vi "Write Value.vi"(8 "error in (no error)":errorcluster, 10 "Value":i64, 11 "int32 in":refnum<class "int64.lvclass">) -> (0 "error out":errorcluster, 3 "int32 out":refnum<class "int64.lvclass">)   [LabVIEW 2020, in "Protobuf RAW.lvlib" / "int64.lvclass"]
uses:
  int64.lvclass
  int64.lvclass/int64.ctl
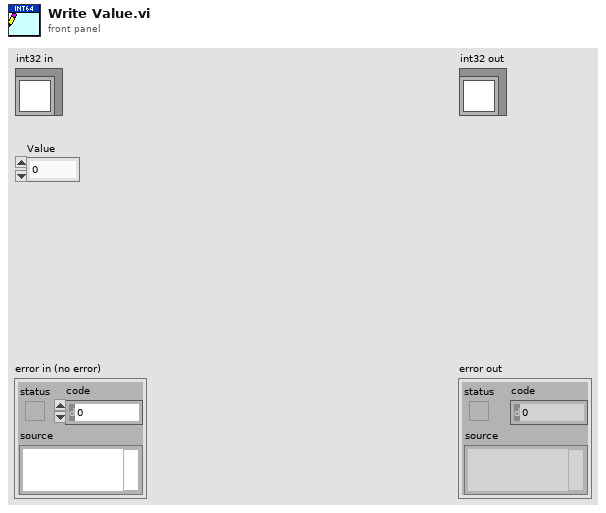
[diagram p1: front panel]
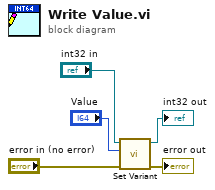
[diagram p0: block diagram]
diagram:
  n1 = call-dynamic "Set Variant.vi"("error in (no error)"="error in (no error)", "Value"="Value", "Proto Type Common in"="int32 in") -> ("error out"=→"error out":errorcluster, "Proto Type Common out"=→"int32 out":refnum<class "int64.lvclass">)  [unwired: 7 in]
